vi "Error Handler - Message Handling Loop.vi"(8 "error in (no error)":errorcluster, 9 "Ignore Errors (Runtime)":i32[](array[numeric]), 10 "Shutdown?":bool=TRUE) -> (0 "dup error in":errorcluster, 2 "Shutdown!":bool, 5 "channel":T1)   [LabVIEW 2023, in "Message Queue Helper.lvlib"]
doc: "Process an error that occurred in the Message Handling Loop, either by ignoring it, or generating an \"Exit\" message."
uses:
  Message Queue Helper.lvlib
  <extravilib>/ChannelInstances/Messenger-t'Message Queue.lvlib-Message Cluster.ctl'/))Channel.ctl
  Message Cluster.ctl
  Enqueue Message.vi
  <extravilib>/ChannelInstances/Messenger-t'Message Queue.lvlib-Message Cluster.ctl'/Write.vi
  <extravilib>/ChannelInstances/Messenger-t'Message Queue.lvlib-Message Cluster.ctl'/Write With Abort.vi
  <extravilib>/ChannelInstances/Messenger-t'Message Queue.lvlib-Message Cluster.ctl'/Endpoint.vi
  Message Queue.lvlib
  <extravilib>/ChannelInstances/Messenger-t'Message Queue.lvlib-Message Cluster.ctl'.lvlib
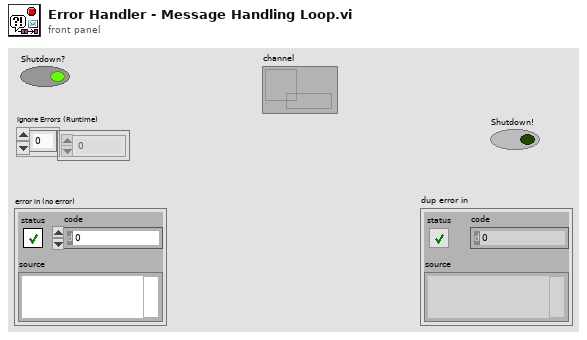
[diagram p1: front panel]
types:
  T1 = typedef "Messenger-t'Message Queue.lvlib-Message Cluster.ctl'.lvlib/))Channel.ctl" = refnum<queue>
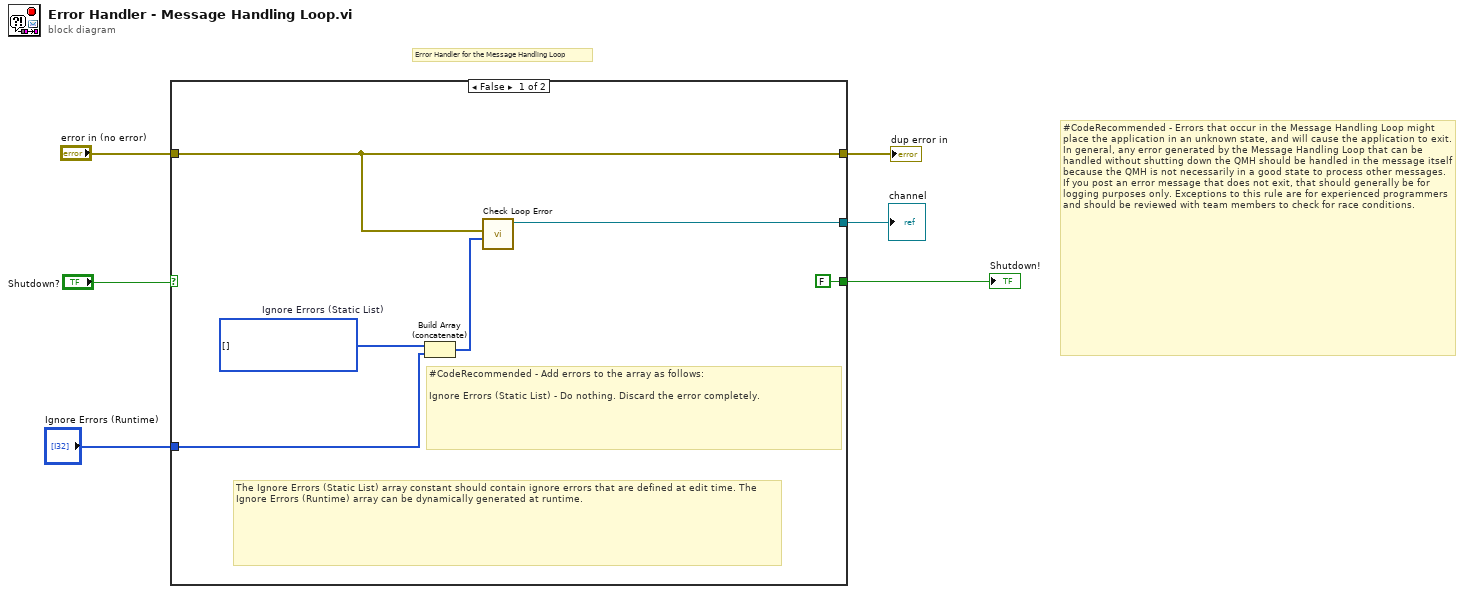
[diagram p0: block diagram]
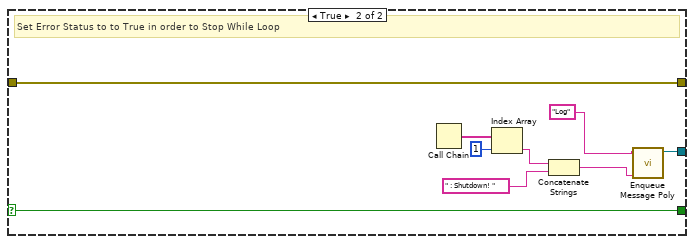
[diagram p2: hidden frame]
diagram:
  # "#CodeRecommended - Errors that occur in the Message Handling Loop might place the application in an unknown state, and will cause the application to exit. In general, any error generated by the Message Handling Loop that can be handled without shutting down the QMH should be handled in the message itself because the QMH is not necessarily in a good state to process other messages. If you post an error message that does not exit, that should generally be for logging purposes only. Exceptions to this rule are for experienced programmers and should be reviewed with team members to check for race conditions."
  # "Error Handler for the Message Handling Loop"
  n1 = case shown="False" "Shutdown?" {
    selector: "Shutdown?" -> [_ w21]
    tunnel: "error in (no error)" -> [w9 w15]
    tunnel: [w10 w19] -> w6
    tunnel: [w9 w15] -> w4
    tunnel: "Ignore Errors (Runtime)" -> [w8 _]
    tunnel: [FALSE w21] -> w1
    frame False {
      w12 = i32[] []  # Ignore Errors (Static List)
      # "The Ignore Errors (Static List) array constant should contain ignore errors that are defined at edit time. The Ignore Errors (Runtime) array can be dynamically generated at runtime."
      # "#CodeRecommended - Add errors to the array as follows:\n\nIgnore Errors (Static List) - Do nothing. Discard the error completely."
      n2 = Build Array (concatenate)(w12, w8) -> (w11:i32[])
      n3 = call "Check Loop Error.vi"("Ignore Errors"=w11, "error to process"=w9) -> ("channel"=w10:T1)  [unwired: 8 in, 1 out]
    }
    frame True {
      # "Set Error Status to to True in order to Stop While Loop"
      n4 = Call Chain() -> (call chain=w16:string[])
      n5 = Index Array(array=w16, index=1) -> (element=w17:string)
      n6 = Concatenate Strings(w17, " : Shutdown! " ("string")) -> (w13:string)
      n7 = call-poly "Enqueue Message Poly.vi"("Message Data"=w13, "Message"="Log" ("message")) -> ("channel"=w19:T1)  [unwired: 9 in]
    }
  }
  "channel" <- w6
  "dup error in" <- w4
  "Shutdown!" <- w1
